vi "Initialize.vi"(0 "VISA Resource Name":refnum<visa-resource-name>="ASRL1", 5 "ID Query? (F: No)":bool, 7 "Device Number (1)":i32=1, 9 "Serial Configuration":T1={"Baud Rate (19200)"=19200, "Flow Control (2: RTS/CTS)"=2, "Parity (2: Even)"=2, "Data Bits (8)"=8, "Stop Bits (20: 2.0)"=20} {"Stop Bits (20: 2.0)" items=["1.0"=10, "1.5"=15, "2.0"=20]; "Data Bits (8)" items=["7"=7, "8"=8]; "Parity (2: Even)" items=["None", "Odd", "Even", "Mark", "Space"]; "Flow Control (2: RTS/CTS)" items=["None"=0, "XON/XOFF"=1, "RTS/CTS"=2, "DTR/DSR"=4]; "Baud Rate (19200)" items=["300"=300, "600"=600, "1200"=1200, "2400"=2400, "4800"=4800, "9600"=9600, "19200"=19200]}, 11 "error in (no error)":errorcluster {"code" format="%.0x"}) -> (4 "VISA Resource Name Out":refnum<visa-resource-name>, 15 "error out":errorcluster {"code" format="%.0x"})   [LabVIEW 2020, in "Olympus IX BX Series.lvlib"]
doc: "This VI passes the addressing information in the instrument decriptor to the Instr Open VI and returns the instrument ID. You can optionally reset the instrument by setting the front panel reset control. You must run this VI before using any of the instrument driver VIs for this instrument.\n\nNote:\n\nVISA library is used to handle all I/O operations with the instrument. All communication parameters can be set through Measurement & Automation Explorer. Default VISA settings are as follows: baud rate 9600, data bits=8, stops bits=1, parity=none, and flow control=none."
uses:
  Olympus IX BX Series.lvlib
panel:
  # "© 2005 National Instruments.  ALL RIGHTS RESERVED."
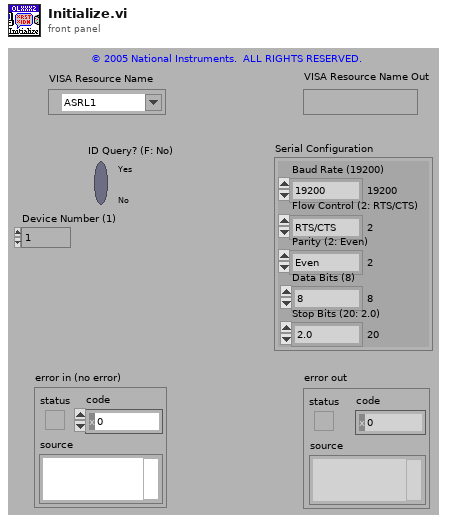
[diagram p1: front panel]
types:
  T1 = cluster{"Baud Rate (19200)":u32, "Flow Control (2: RTS/CTS)":u16, "Parity (2: Even)":u16, "Data Bits (8)":u16, "Stop Bits (20: 2.0)":u16}
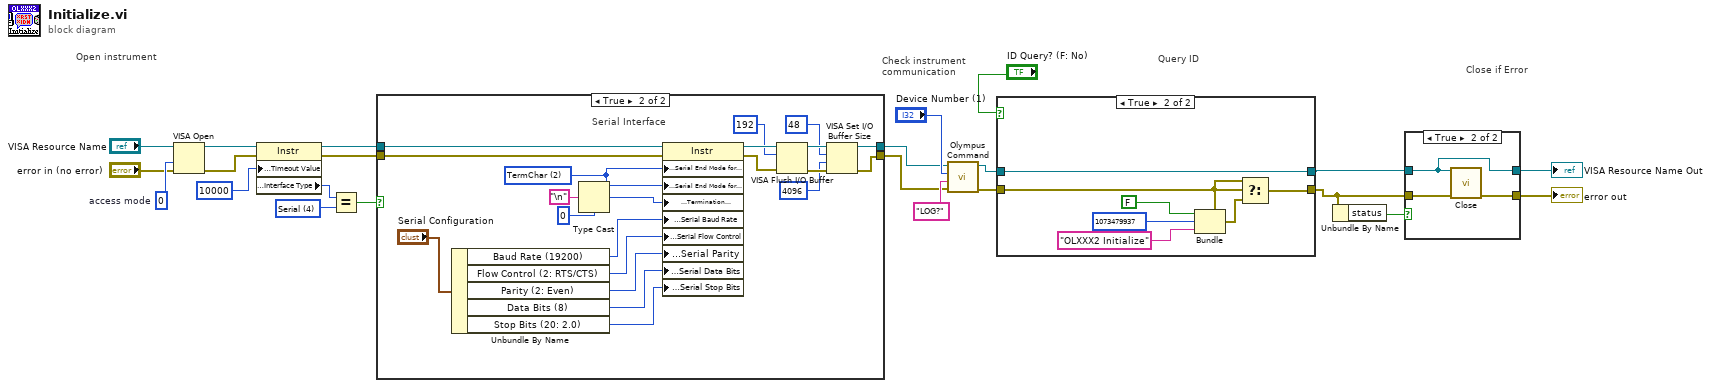
[diagram p0: block diagram]
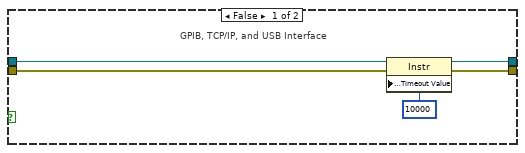
[diagram p3: hidden frame]
diagram:
  w19 = u32 0  # access mode
  w18 = u16 4 items=["GPIB"=1, "VXI"=2, "GPIB-VXI"=3, "Serial"=4, "PXI"=5, "TCPIP"=6, "USB"=7] ("Interface Information:Interface Type")
  # "Check instrument\ncommunication"
  # "Close if Error"
  # "Query ID"
  # "Open instrument"
  n1 = VISA Open(access mode=w19, error in (no error)="error in (no error)", VISA resource name="VISA Resource Name") -> (VISA resource name=w3:refnum<visa-resource-name>, error out=w4:errorcluster)  [unwired: 2 in]
  n2 = property class="Instr"(reference=w3, error in=w4, "General Settings:Timeout Value"=u32 10000) -> (reference out=w13:refnum<visa-resource-name>, error out=w12:errorcluster, "Interface Information:Interface Type"=w16:u16)
  n3 = Equal?(x=w16, y=w18) -> (x = y?=w11:bool)
  n4 = case shown="True" w11 {
    tunnel: [w27 w46] -> w10
    tunnel: [w26 w43] -> w9
    tunnel: w13 -> [w25 w48]
    tunnel: w12 -> [w24 w49]
    frame False {
      # "GPIB, TCP/IP, and USB Interface"
      n5 = property class="Instr"(reference=w25, error in=w24, "General Settings:Timeout Value"=u32 10000 ("Tmo Value")) -> (reference out=w27:refnum<visa-resource-name>, error out=w26:errorcluster)
    }
    frame True {
      w36 = u16 2 items=["None", "LastBit", "TermChar"] ("Serial Settings:Serial End Mode for Reads")
      # "Serial Interface"
      n6 = Unbundle By Name("Serial Configuration") -> ("Baud Rate (19200)"=w33:u32, "Flow Control (2: RTS/CTS)"=w32:u16, "Parity (2: Even)"=w29:u16, "Data Bits (8)"=w31:u16, "Stop Bits (20: 2.0)"=w30:u16)
      n7 = Type Cast(type=u8 0, x="\n" ("Line Feed Constant")) -> (*(type *) &x=w35:u8)
      n8 = property class="Instr"(reference=w48, error in=w49, "Serial Settings:Serial End Mode for Reads"=w36, "Serial Settings:Serial End Mode for Writes"=w36, "Message Based Settings:Termination Character"=w35, "Serial Settings:Serial Baud Rate"=w33, "Serial Settings:Serial Flow Control"=w32, "Serial Settings:Serial Parity"=w29, "Serial Settings:Serial Data Bits"=w31, "Serial Settings:Serial Stop Bits"=w30) -> (reference out=w42:refnum<visa-resource-name>, error out=w45:errorcluster)
      n9 = VISA Flush I/O Buffer(VISA resource name=w42, mask (16)=u16 192, error in (no error)=w45) -> (VISA resource name out=w47:refnum<visa-resource-name>, error out=w44:errorcluster)
      n10 = VISA Set I/O Buffer Size(VISA resource name=w47, mask (16)=u16 48, size (4096)=u32 4096 ("size (0)"), error in (no error)=w44) -> (VISA resource name out=w46:refnum<visa-resource-name>, error out=w43:errorcluster)
    }
  }
  n11 = call "Olympus Command.vi"("error in (no error)"=w9, "Command string"="LOG?", "Device Number (1)"="Device Number (1)", "VISA Resource Name"=w10) -> ("error out"=w22:errorcluster, "VISA Resource Name Out"=w23:refnum<visa-resource-name>)  [unwired: 5 in, 1 out]
  n12 = case shown="True" "ID Query? (F: No)" {
    tunnel: [w51 w55] -> w2
    tunnel: w23 -> [w51 w55]
    tunnel: [w50 w53] -> w1
    tunnel: w22 -> [w50 w52]
    frame False {
    }
    frame True {
      n13 = Bundle(cluster=w52, "status"=FALSE, "code"=1073479937, "source"="OLXXX2 Initialize" ("regular expression")) -> (w54:errorcluster)
      n14 = Select(t=w52, s=w52, f=w54) -> (s? t:f=w53:errorcluster)
    }
  }
  n15 = Unbundle By Name(w1) -> ("status"=w8:bool)
  n16 = case shown="True" w8 {
    tunnel: w1 -> [w59 w63]
    tunnel: w2 -> [w60 w61]
    tunnel: [w60 w61] -> w7
    tunnel: [w59 w62] -> w6
    frame False {
    }
    frame True {
      n17 = call "Close.vi"("VISA Resource Name"=w61, "error in (no error)"=w63) -> ("error out"=w62:errorcluster)  [unwired: 13 in]
    }
  }
  "VISA Resource Name Out" <- w7
  "error out" <- w6
